vi "Check if Channels Present.vi"(8 "error in (no error)":errorcluster, 9 "Channel Names":string[](array[string]), 10 "Group name":string, 11 "Refnum in":refnum<k34>) -> (0 "error out":errorcluster, 2 "Passed ?":bool, 3 "Refnum out":refnum<k34>)   [LabVIEW 2026, in "Telemetry System Tests.lvclass"]
uses:
  Telemetry System Tests.lvclass
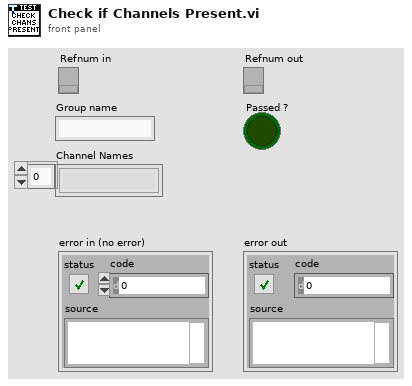
[diagram p1: front panel]
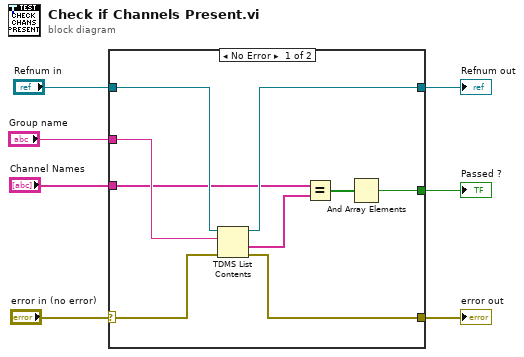
[diagram p0: block diagram]
diagram:
  n1 = case shown="No Error" "error in (no error)" {
    selector: "error in (no error)" -> [w8 w17]
    tunnel: "Group name" -> [w16 _]
    tunnel: [w15 w18] -> w6
    tunnel: [w14 w17] -> w5
    tunnel: "Refnum in" -> [w13 w18]
    tunnel: "Channel Names" -> [w12 _]
    tunnel: [w9 _] -> w2
    frame No Error {
      n2 = TDMS List Contents(4:w8, 6:w16, 7:w13) -> (0:w14:errorcluster, 1:w11:string[], 3:w15:refnum<k34>)  [unwired: 1 out]
      n3 = Equal?(x=w12, y=w11) -> (x = y?=w10:bool[])
      n4 = And Array Elements(Boolean array=w10) -> (logical AND=w9:bool)
    }
    frame Error {
    }
  }
  "Refnum out" <- w6
  "error out" <- w5
  "Passed ?" <- w2
